vi "Test LV2.vi"(0 "Ref In":refnum<vi>, 11 "error in (no error)":errorcluster, 13 "Operation":T1) -> (4 "Ref Out":refnum<vi>, 15 "error out":errorcluster)   [LabVIEW 2016, in "Drona Path obtn.lvlib"]
uses:
  Drona Path obtn.lvlib
  Typedefs/Test LV2 Enum.ctl
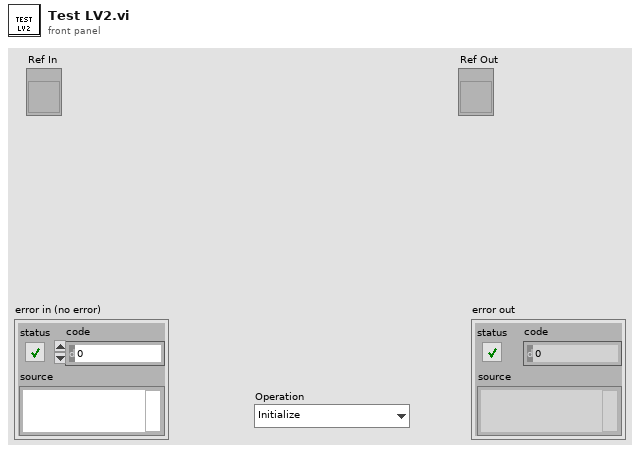
[diagram p1: front panel]
types:
  T1 = typedef "Drona Path obtn.lvlib/Test LV2 Enum.ctl" = enum16{"Initialize", "Write", "Read"}
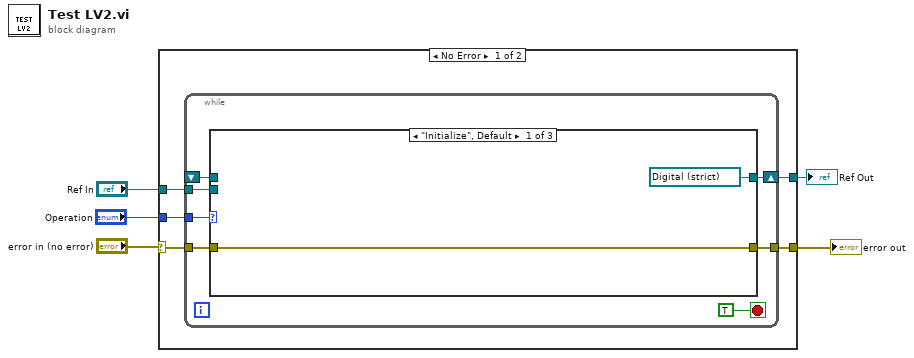
[diagram p0: block diagram]
diagram:
  n1 = case shown="No Error" "error in (no error)" {
    selector: "error in (no error)" -> [w10 w24]
    tunnel: [w9 w24] -> w4
    tunnel: "Operation" -> [w8 _]
    tunnel: "Ref In" -> [w7 w25]
    tunnel: [w6 w25] -> w1
    frame No Error {
      n2 = while {
        tunnel: w10 -> [w16]
        tunnel: [w17] -> w9
        tunnel: w8 -> [w15]
        tunnel: w7 -> [w13]
        shift-right: [w12] -> w6
        shift-left: _ -> [w11]
        stop <- TRUE stop-if-true
        n3 = case shown="\"Initialize\", Default" w15 {
          tunnel: [w19 w21 w23] -> w17
          tunnel: w16 -> [w19 w21 w23]
          tunnel: w13 -> [_ w20 _]
          tunnel: [refnum<vi> refnum ("Ref In") w20 w22] -> w12
          tunnel: w11 -> [_ _ w22]
          frame "Initialize", Default {
          }
          frame "Write" {
          }
          frame "Read" {
          }
        }
      }
    }
    frame Error {
    }
  }
  "error out" <- w4
  "Ref Out" <- w1
